vi "Get Column Names.vi"(8 "error in (no error)":errorcluster, 9 "tableName":string, 10 "schema":string, 11 "Post Analysis in":refnum<class "Post Analysis.lvclass">) -> (0 "error out":errorcluster, 1 "columnNamesForQuery":string[](array[string]), 2 "columnNames":string[](array[string]), 3 "Post Analysis out":refnum<class "Post Analysis.lvclass">)   [LabVIEW 2023, in "Data Analysis.lvlib" / "Post Analysis.lvlib" / "Post Analysis.lvclass"]
uses:
  Post Analysis.lvclass
  Post Analysis.lvclass/Post Analysis.ctl
  HardwareAbstractionLayer_LVOOP/Database/Database.lvclass
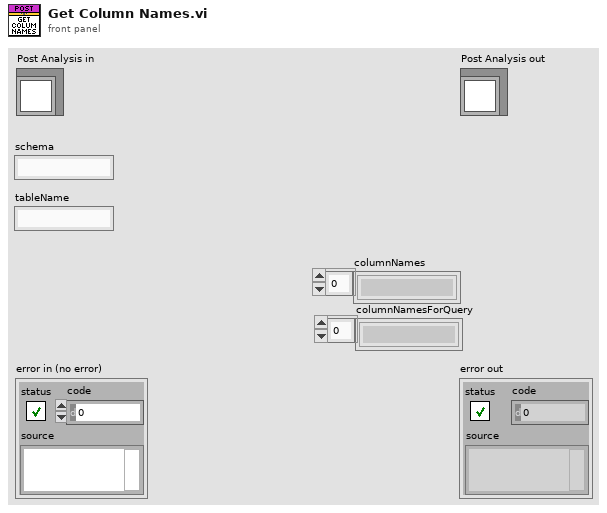
[diagram p1: front panel]
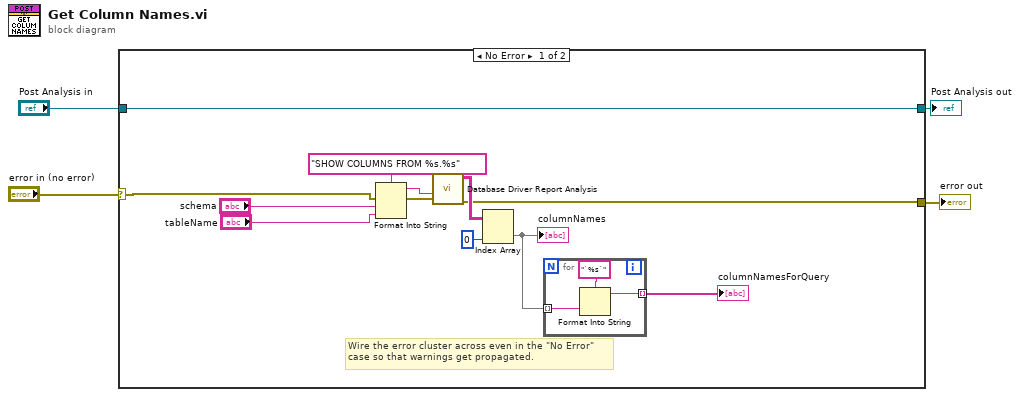
[diagram p0: block diagram]
diagram:
  n1 = case shown="No Error" "error in (no error)" {
    selector: "error in (no error)" -> [w6 w21]
    tunnel: [w5 w21] -> w3
    tunnel: [w16 w20] -> w1
    tunnel: "Post Analysis in" -> [w16 w20]
    frame No Error {
      # "Wire the error cluster across even in the \"No Error\"\ncase so that warnings get propagated."
      n2 = Format Into String(format string="SHOW COLUMNS FROM %s.%s" ("SQL query"), error in=w6, "schema", "tableName") -> (resulting string=w12:string, error out=w11:errorcluster)  [unwired: 1 in]
      n3 = call "Database Driver Report Analysis.vi"("error in"=w11, "SQL query"=w12) -> ("error out"=w5:errorcluster, "data"=w13:string[][])  [unwired: 6 in, 2 out]
      n4 = Index Array(array=w13, index (col)=0 ("disabled index (col)")) -> (element=w8:string[])  [unwired: 1 in]
      "columnNames" <- w8
      n5 = for {
        tunnel: w8 -> [w19] mode=indexing
        tunnel: [w17] -> w7 mode=indexing
        n6 = Format Into String(format string="`%s`", w19) -> (resulting string=w17:string)  [unwired: 2 in, 1 out]
      }
      "columnNamesForQuery" <- w7
    }
    frame Error {
    }
  }
  "error out" <- w3
  "Post Analysis out" <- w1
